vi "Initialize from PS.vi"(8 "error in (no error)":errorcluster, 11 "PS Driver AMI4xx in":refnum<class "PS Driver AMI4xx.lvclass">) -> (0 "error out":errorcluster, 2 "PS Values":T1, 3 "PS Driver AMI4xx out":refnum<class "PS Driver AMI4xx.lvclass">)   [LabVIEW 2025, in "PS Driver.lvlib" / "PS Driver AMI4xx.lvclass"]
doc: "Author: Scott Hannahs <sth@magnet.fsu.edu>\n\nThis software is licensed for use under the “MIT License\"\nCopyright (c) 2025 Scott Hannahs, sth@sth@magnet.sthnet.net\n\nPermission is hereby granted, free of charge, to any person obtaining a copy of this software and associated documentation files (the \"Software\"), to deal in the Software without restriction, including without limitation the rights to use, copy, modify, merge, publish, distribute, sublicense, and/or sell copies of the Software, and to permit persons to whom the Software is furnished to do so, subject to the following conditions: The above copyright notice and this permission notice shall be included in all copies or substantial portions of the Software.\n\nTHE SOFTWARE IS PROVIDED \"AS IS\", WITHOUT WARRANTY OF ANY KIND, EXPRESS OR IMPLIED, INCLUDING BUT NOT LIMITED TO THE WARRANTIES OF MERCHANTABILITY, FITNESS FOR A PARTICULAR PURPOSE AND NONINFRINGEMENT. IN NO EVENT SHALL THE AUTHORS OR COPYRIGHT HOLDERS BE LIABLE FOR ANY CLAIM, DAMAGES OR OTHER LIABILITY, WHETHER IN AN ACTION OF CONTRACT, TORT OR OTHERWISE, ARISING FROM, OUT OF OR IN CONNECTION WITH THE SOFTWARE OR THE USE OR OTHER DEALINGS IN THE SOFTWARE."
uses:
  PS Driver AMI4xx.lvclass
  PS Driver with Persistence.lvclass
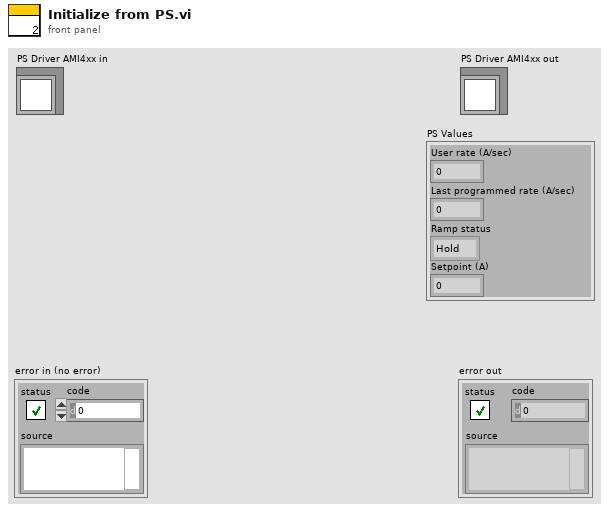
[diagram p1: front panel]
types:
  T1 = cluster{"User rate (A/sec)":dbl, "Last programmed rate (A/sec)":dbl, "Ramp status":enum16{"Hold", "Ramp to zero", "Ramp to setpoint"}, "Setpoint (A)":dbl}
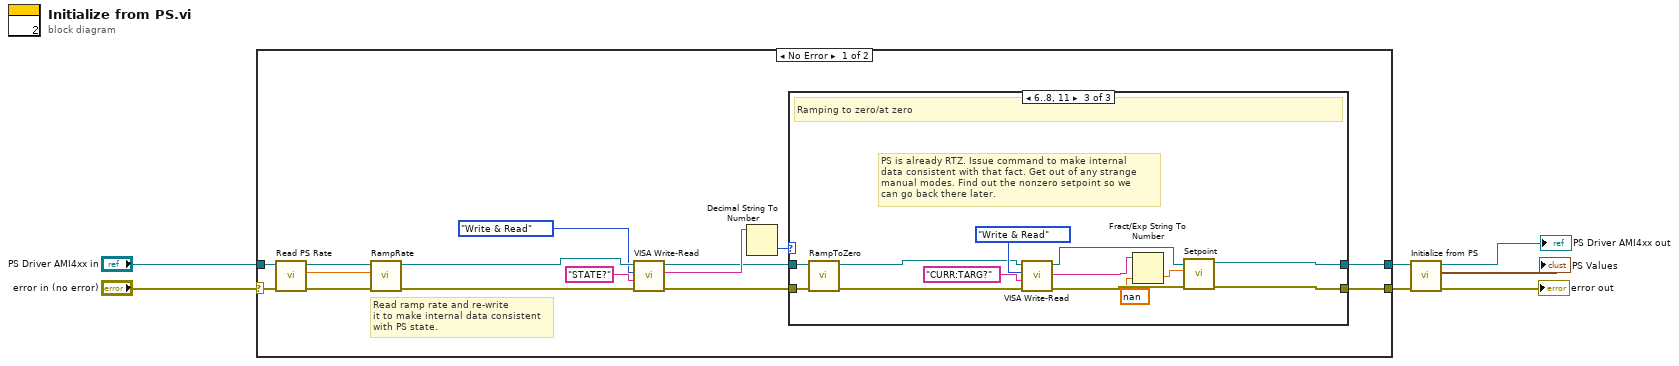
[diagram p0: block diagram]
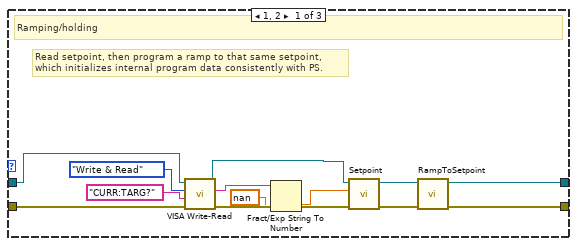
[diagram p2: hidden frame]
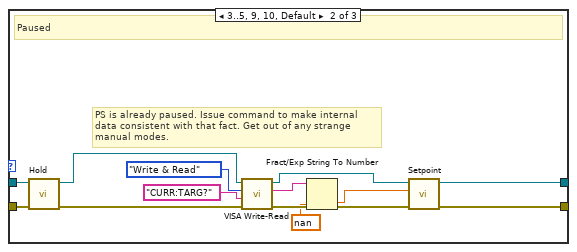
[diagram p3: hidden frame]
diagram:
  n1 = case shown="No Error" "error in (no error)" {
    selector: "error in (no error)" -> [w21 w62]
    tunnel: [w8 w62] -> w4
    tunnel: [w9 w63] -> w5
    tunnel: "PS Driver AMI4xx in" -> [w22 w63]
    frame No Error {
      # "Read ramp rate and re-write\nit to make internal data consistent\nwith PS state."
      n2 = call-dynamic "Read PS Rate.vi"("error in (no error)"=w21, "PS Driver AMI4xx in"=w22) -> ("error out"=w20:errorcluster, "Ramp rate (A/s)"=w18:dbl, "PS Driver AMI4xx out"=w19:refnum<class "PS Driver AMI4xx.lvclass">)  [unwired: 7 in]
      n3 = call-dynamic "RampRate.vi"("error in (no error)"=w20, "Ramp rate (A/s)"=w18, "PS Driver AMI4xx in"=w19) -> ("error out"=w15:errorcluster, "PS Driver AMI4xx out"=w17:refnum<class "PS Driver AMI4xx.lvclass">)  [unwired: 6 in, 1 out]
      n4 = call "VISA Write-Read.vi"("error in (no error)"=w15, "Command String"="STATE?", "Action"=enum16{"Write", "Read", "Write & Read"}."Write & Read", "PS Driver.lvlib:PS Driver AMI4xx.lvclass"=w17) -> ("error out"=w10:errorcluster, "Response string"=w13:string, "PS Driver.lvlib:PS Driver AMI4xx.lvclass out"=w11:refnum<class "PS Driver AMI4xx.lvclass">)  [unwired: 4 in, 1 out]
      n5 = Decimal String To Number(string=w13) -> (number=w12:i32)  [unwired: 2 in, 1 out]
      n6 = case shown="6..8, 11" w12 {
        tunnel: w11 -> [w33 w48 w54]
        tunnel: w10 -> [w32 w47 w53]
        tunnel: [w24 w38 w50] -> w9
        tunnel: [w23 w39 w49] -> w8
        frame 1, 2 {
          # "Read setpoint, then program a ramp to that same setpoint,\nwhich initializes internal program data consistently with PS."
          # "Ramping/holding"
          n7 = call "VISA Write-Read.vi"("error in (no error)"=w32, "Command String"="CURR:TARG?", "Action"=enum16{"Write", "Read", "Write & Read"}."Write & Read", "PS Driver.lvlib:PS Driver AMI4xx.lvclass"=w33) -> ("error out"=w29:errorcluster, "Response string"=w31:string, "PS Driver.lvlib:PS Driver AMI4xx.lvclass out"=w30:refnum<class "PS Driver AMI4xx.lvclass">)  [unwired: 4 in, 1 out]
          n8 = Fract/Exp String To Number(string=w31, default (0 dbl)=nan ("default (0 DBL)")) -> (number=w28:dbl)  [unwired: 2 in, 1 out]
          n9 = call-dynamic "Setpoint.vi"("error in (no error)"=w29, "Setpoint [A]"=w28, "PS Driver AMI4xx.lvlib:PS Driver AMI4xx.lvclass in"=w30) -> ("error out"=w25:errorcluster, "PS Driver AMI4xx.lvlib:PS Driver AMI4xx.lvclass out"=w26:refnum<class "PS Driver AMI4xx.lvclass">)  [unwired: 6 in, 1 out]
          n10 = call-dynamic "RampToSetpoint.vi"("error in (no error)"=w25, "PS Driver AMI4xx.lvlib:PS Driver AMI4xx.lvclass in"=w26) -> ("error out"=w23:errorcluster, "PS Driver AMI4xx.lvlib:PS Driver AMI4xx.lvclass out"=w24:refnum<class "PS Driver AMI4xx.lvclass">)  [unwired: 8 in]
        }
        frame 3..5, 9, 10, Default {
          # "PS is already paused. Issue command to make internal\ndata consistent with that fact. Get out of any strange\nmanual modes."
          # "Paused"
          n11 = call-dynamic "Hold.vi"("error in (no error)"=w47, "PS Driver AMI4xx.lvlib:PS Driver AMI4xx.lvclass in"=w48) -> ("error out"=w36:errorcluster, "PS Driver AMI4xx.lvlib:PS Driver AMI4xx.lvclass out"=w37:refnum<class "PS Driver AMI4xx.lvclass">)  [unwired: 8 in]
          n12 = call "VISA Write-Read.vi"("error in (no error)"=w36, "Command String"="CURR:TARG?", "Action"=enum16{"Write", "Read", "Write & Read"}."Write & Read", "PS Driver.lvlib:PS Driver AMI4xx.lvclass"=w37) -> ("error out"=w42:errorcluster, "Response string"=w44:string, "PS Driver.lvlib:PS Driver AMI4xx.lvclass out"=w43:refnum<class "PS Driver AMI4xx.lvclass">)  [unwired: 4 in, 1 out]
          n13 = Fract/Exp String To Number(string=w44, default (0 dbl)=nan ("default (0 DBL)")) -> (number=w41:dbl)  [unwired: 2 in, 1 out]
          n14 = call-dynamic "Setpoint.vi"("error in (no error)"=w42, "Setpoint [A]"=w41, "PS Driver AMI4xx.lvlib:PS Driver AMI4xx.lvclass in"=w43) -> ("error out"=w39:errorcluster, "PS Driver AMI4xx.lvlib:PS Driver AMI4xx.lvclass out"=w38:refnum<class "PS Driver AMI4xx.lvclass">)  [unwired: 6 in, 1 out]
        }
        frame 6..8, 11 {
          # "PS is already RTZ. Issue command to make internal\ndata consistent with that fact. Get out of any strange\nmanual modes. Find out the nonzero setpoint so we \ncan go back there later."
          # "Ramping to zero/at zero"
          n15 = call-dynamic "RampToZero.vi"("error in (no error)"=w53, "PS Driver AMI4xx.lvlib:PS Driver AMI4xx.lvclass in"=w54) -> ("error out"=w52:errorcluster, "PS Driver AMI4xx.lvlib:PS Driver AMI4xx.lvclass out"=w51:refnum<class "PS Driver AMI4xx.lvclass">)  [unwired: 8 in]
          n16 = call "VISA Write-Read.vi"("error in (no error)"=w52, "Command String"="CURR:TARG?", "Action"=enum16{"Write", "Read", "Write & Read"}."Write & Read", "PS Driver.lvlib:PS Driver AMI4xx.lvclass"=w51) -> ("error out"=w57:errorcluster, "Response string"=w59:string, "PS Driver.lvlib:PS Driver AMI4xx.lvclass out"=w58:refnum<class "PS Driver AMI4xx.lvclass">)  [unwired: 4 in, 1 out]
          n17 = Fract/Exp String To Number(string=w59, default (0 dbl)=nan ("default (0 DBL)")) -> (number=w56:dbl)  [unwired: 2 in, 1 out]
          n18 = call-dynamic "Setpoint.vi"("error in (no error)"=w57, "Setpoint [A]"=w56, "PS Driver AMI4xx.lvlib:PS Driver AMI4xx.lvclass in"=w58) -> ("error out"=w49:errorcluster, "PS Driver AMI4xx.lvlib:PS Driver AMI4xx.lvclass out"=w50:refnum<class "PS Driver AMI4xx.lvclass">)  [unwired: 6 in, 1 out]
        }
      }
    }
    frame Error {
    }
  }
  n19 = call-parent "Initialize from PS.vi"("error in (no error)"=w4, "PS Driver in"=w5) -> ("error out"=→"error out":errorcluster, "PS Values"=→"PS Values":T1, "PS Driver out"=→"PS Driver AMI4xx out":refnum<class "PS Driver AMI4xx.lvclass">)  [unwired: 7 in]
